vi "Control Pivot Left.vi"   [LabVIEW 2020]
uses:
  Framework/Robot Global Data.vi
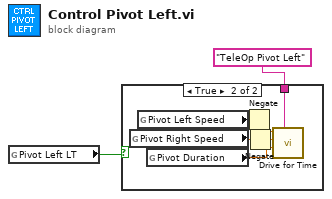
[diagram p0: block diagram]
diagram:
  n1 = global read "Robot Global Data.vi" "Pivot Left LT"() -> (w2:bool)
  n2 = case shown="True" w2 {
    tunnel: "TeleOp Pivot Left" ("Description") -> [_ w8]
    frame False {
    }
    frame True {
      n3 = global read "Robot Global Data.vi" "Pivot Right Speed"() -> (w6:dbl)
      n4 = global read "Robot Global Data.vi" "Pivot Left Speed"() -> (w7:dbl)
      n5 = global read "Robot Global Data.vi" "Pivot Duration"() -> (w5:dbl)
      n6 = Negate(x=w7) -> (-x=w4:dbl)
      n7 = Negate(x=w6) -> (-x=w3:dbl)
      n8 = call "Drive for Time.vi"("Description"=w8, "Seconds"=w5, "Right Speed"=w3, "Left Speed"=w4) -> ()  [unwired: 7 in, 1 out]
    }
  }
